vi "4431 Sensor Inputs.vi"(3 "error in":errorcluster, 4 "Enum":enum16{"RS232", "LED", "BEEPER", "PAGER"}(ring)) -> (0 "error out":errorcluster, 1 "Numeric":dbl)   [LabVIEW 2014]
panel:
  out "Numeric 2":dbl
  out "Waveform Graph":dynamicdata(graph)
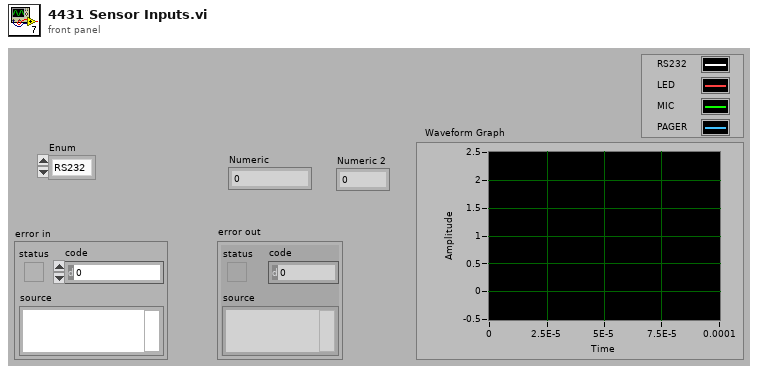
[diagram p1: front panel]
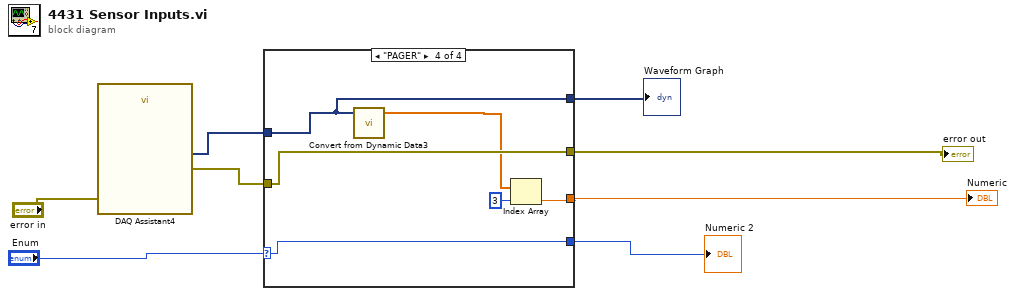
[diagram p0: block diagram]
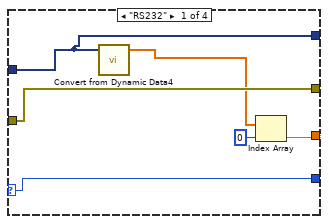
[diagram p2: hidden frame]
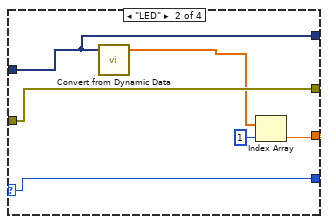
[diagram p3: hidden frame]
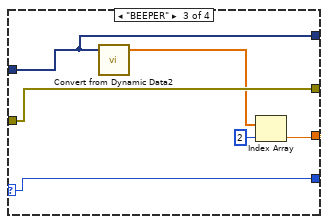
[diagram p4: hidden frame]
diagram:
  n1 = call "DAQ Assistant4"("error in"="error in") -> ("data"=w3:dynamicdata, "error out"=w4:errorcluster)  [unwired: 16 in, 1 out]
  n2 = case shown="\"PAGER\"" "Enum" {
    selector: "Enum" -> [w11 w17 w23 w29]
    tunnel: w4 -> [w13 w19 w25 w31]
    tunnel: [w13 w19 w25 w31] -> w8
    tunnel: [w14 w20 w26 w32] -> w6
    tunnel: w3 -> [w12 w18 w24 w30]
    tunnel: [w12 w18 w24 w30] -> w2
    tunnel: [w11 w17 w23 w29] -> w1
    frame "RS232" {
      n3 = call "Convert from Dynamic Data4"("Dynamic Data Type"=w12) -> ("Array"=w9:dbl[])  [unwired: 3 in]
      n4 = Index Array(array=w9, index=0) -> (element=w14:dbl)
    }
    frame "LED" {
      n5 = call "Convert from Dynamic Data"("Dynamic Data Type"=w18) -> ("Array"=w15:dbl[])  [unwired: 3 in]
      n6 = Index Array(array=w15, index=1) -> (element=w20:dbl)
    }
    frame "BEEPER" {
      n7 = call "Convert from Dynamic Data2"("Dynamic Data Type"=w24) -> ("Array"=w21:dbl[])  [unwired: 3 in]
      n8 = Index Array(array=w21, index=2) -> (element=w26:dbl)
    }
    frame "PAGER" {
      n9 = call "Convert from Dynamic Data3"("Dynamic Data Type"=w30) -> ("Array"=w27:dbl[])  [unwired: 3 in]
      n10 = Index Array(array=w27, index=3) -> (element=w32:dbl)
    }
  }
  "error out" <- w8
  "Numeric" <- w6
  "Waveform Graph" <- w2
  "Numeric 2" <- w1
